vi "Configure Trigger Source and Mode.vi"(6 "Settle (1mS)":u32=1, 7 "Trigger Delay (0)":dbl min=0.0 max=65.0 step=0.001 format="%_4g", 8 "error in (no error)":errorcluster, 9 "Trigger Out Mode (0: Off)":u16(ring) items=["Off", "Trigger", "FSTR"], 10 "Trigger  Source (0: External)":u16(ring) items=["External", "Bus"], 11 "VISA resource name":refnum<visa-resource-name>) -> (0 "error out":errorcluster, 3 "VISA resource name out":refnum<visa-resource-name>)   [LabVIEW 2012, in "TDK-Lambda Z.lvlib"]
doc: "Selects the power supply input trigger source as follows:\n Bus - (*TRG & TRIG) and Front Panel \nExternal - Mainframe backplane Trigger In Pin\nSets the time delay between the detection of an event on the specified trigger source and the start of any corresponding trigger action on the power supply's output.\nSets the operation of the Trigger Out signal to either Off Function Strobe or Trigger mode. Factory default is Off.\n\nNote: This VI will wait for \"Settle\" milliseconds after setting the limit to allow the output to reach the new setting. If unwired, there will be no delay"
uses:
  TDK-Lambda Z.lvlib
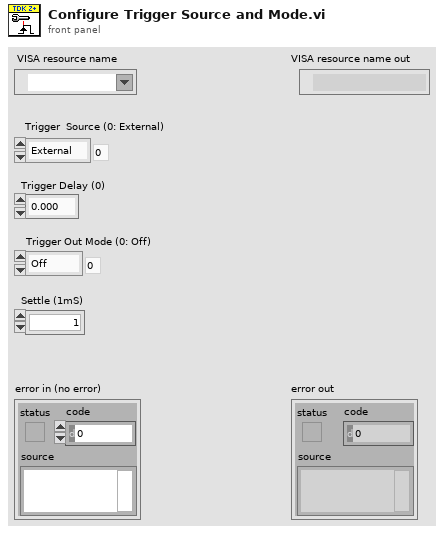
[diagram p1: front panel]
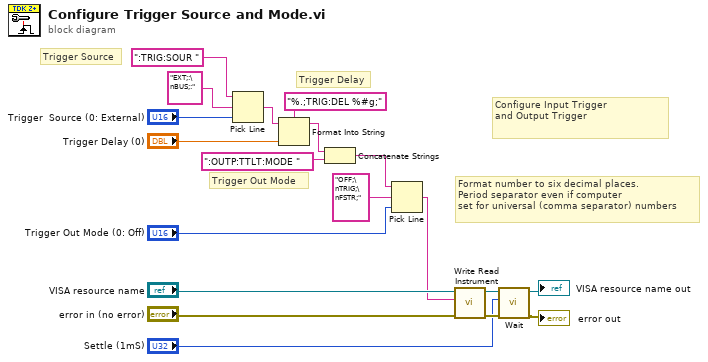
[diagram p0: block diagram]
diagram:
  # "Configure Input Trigger \nand Output Trigger"
  # "Trigger Out Mode"
  # "Trigger Delay"
  # "Trigger Source"
  # "Format number to six decimal places.\nPeriod separator even if computer \nset for universal (comma separator) numbers"
  n1 = Pick Line(string ("")=":TRIG:SOUR " ("format string"), multi-line string="EXT;:\nBUS;:" ("format string"), line index="Trigger  Source (0: External)") -> (output string=w8:string)
  n2 = Format Into String(format string="%.;TRIG:DEL %#g;", initial string=w8, "Trigger Delay (0)") -> (resulting string=w4:string)  [unwired: 1 in, 1 out]
  n3 = Concatenate Strings(w4, ":OUTP:TTLT:MODE " ("string")) -> (w3:string)
  n4 = Pick Line(string ("")=w3, multi-line string="OFF;\nTRIG;\nFSTR;" ("format string"), line index="Trigger Out Mode (0: Off)") -> (output string=w1:string)
  n5 = call "Write Read Instrument.vi"("error in (no error)"="error in (no error)", "SCPI  Write Command/Query"=w1, "VISA resource name"="VISA resource name") -> ("error out"=w16:errorcluster, "VISA resource name out"=w17:refnum<visa-resource-name>)  [unwired: 6 in, 1 out]
  n6 = call "Wait.vi"("error in (no error)"=w16, "Wait (1mS)"="Settle (1mS)", "VISA resource name"=w17) -> ("error out"=→"error out":errorcluster, "VISA resource name out"=→"VISA resource name out":refnum<visa-resource-name>)  [unwired: 7 in]
